vi "accelerometer zero panel.vi"(8 "error in (no error)":errorcluster, 11 "disk queues":T1) -> (0 "error out":errorcluster, 1 "yzero":dbl, 2 "xzero":dbl, 3 "set":bool)   [LabVIEW 2017]
uses:
  typedefs/queue cluster.ctl
  typedefs/reading queue.ctl
  typedefs/reading.ctl
  typedefs/readingType.ctl
  typedefs/reading1.ctl
  <vilib>/Analysis/baseanly.llb/Mean (DBL).vi
  <vilib>/Analysis/NI_AALBase.lvlib
panel:
  in  "cancel":bool
  in  "add reading":bool
  out "accel range":T3
  in  "reset":bool
  in  "Set Acceleromter Zero":bool
  out "Ya":dbl(slide) scale=-1.0..1.0 scale format="%#.2f"
  out "Xa":dbl(slide) scale=-1.0..1.0 scale format="%#.2f"
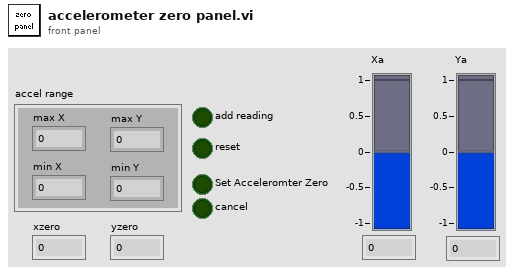
[diagram p1: front panel]
types:
  T1 = typedef "queue cluster.ctl" = cluster{"voltage":T2, "coil":T2, "mag":T2, "accel":T2, "slope":refnum<queue>, "angle":refnum<queue>}
  T2 = typedef "reading queue.ctl" = refnum<queue>
  T3 = cluster{"max X":dbl, "min X":dbl, "max Y":dbl, "min Y":dbl}
  T4 = typedef "reading.ctl" = cluster{"reading type":T5, "time":fxp<+,48,48>, "x":sgl, "y":sgl, "z":sgl, "XSUM":u8}
  T5 = typedef "readingType.ctl" = enum8{"SYNC", "DETVAL", "COILI", "MAGVEC", "ACCVEC"}
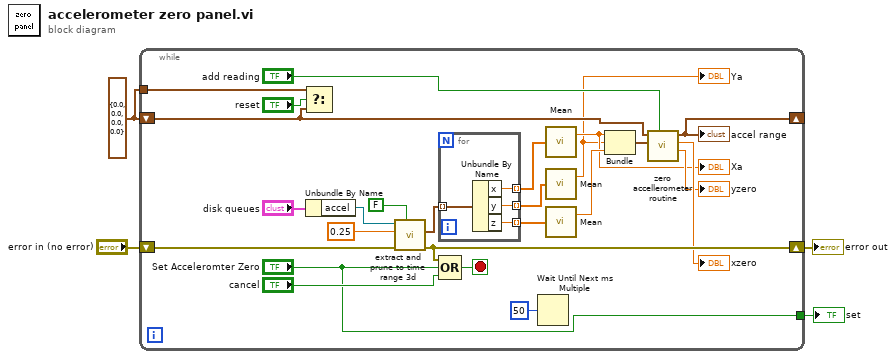
[diagram p0: block diagram]
diagram:
  w4 = T3 {"max X"=0.0, "min X"=0.0, "max Y"=0.0, "min Y"=0.0} ("accel range out")
  n1 = while {
    shift-right: [w18] -> _
    shift-left: w4 -> [w16]
    tunnel: w4 -> [w15]
    shift-right: [w11] -> w2
    shift-left: "error in (no error)" -> [w12]
    tunnel: ["Set Acceleromter Zero"] -> w1
    stop <- w13 stop-if-true
    n2 = Select(t=w15, s="reset", f=w16) -> ()  [unwired: 1 out]
    n3 = Unbundle By Name("disk queues") -> ("accel"=w28:T2)
    n4 = call "extract and prune to time range 3d.vi"("prune?"=FALSE, "error in (no error)"=w12, "time range (s)"=0.25 ("time range"), "queue in"=w28) -> ("error out"=w11:errorcluster, "extracted data"=w25:T4[])  [unwired: 4 in, 2 out]
    n5 = for {
      tunnel: w25 -> [w33] mode=indexing
      tunnel: [w32] -> w24 mode=indexing
      tunnel: [w31] -> w23 mode=indexing
      tunnel: [w30] -> w22 mode=indexing
      n6 = Unbundle By Name(w33) -> ("x"=w32:sgl, "y"=w31:sgl, "z"=w30:sgl)
    }
    n7 = Compound Arithmetic op=OR(w11, "Set Acceleromter Zero", "cancel") -> (w13:bool)
    n8 = Wait Until Next ms Multiple(millisecond multiple=u32 50) -> ()  [unwired: 1 out]
    n9 = call-poly <vilib>:"Mean.vi"("X"=w24) -> ("mean"=w8:dbl)  [unwired: 1 out]
    "Xa" <- w8
    n10 = call-poly <vilib>:"Mean.vi"("X"=w23) -> ("mean"=w7:dbl)  [unwired: 1 out]
    "Ya" <- w7
    n11 = call-poly <vilib>:"Mean.vi"("X"=w22) -> ("mean"=w21:dbl)  [unwired: 1 out]
    n12 = Bundle("mean"=w8, "mean"=w7, "mean"=w21) -> (w20:cluster{"mean":dbl, "mean":dbl, "mean":dbl})  [unwired: 1 in]
    n13 = call "zero accellerometer routine.vi"("add reading"="add reading", "accel"=w20, "accel range"=w16) -> ("y offset"=→"yzero":dbl, "x offset"=→"xzero":dbl, "accel range out"=w18:T3)  [unwired: 6 in]
    "accel range" <- w18
  }
  "error out" <- w2
  "set" <- w1
